vi "Set Data Value.vi"(8 "error in (no error)":errorcluster, 9 "Flat Data":u8[](array[numeric]) format="%.0x", 11 "CIFTag in":refnum<class "CIF_CIPC_Chn_String.lvclass">) -> (0 "error out":errorcluster, 1 "Updated":bool, 3 "CIFTag out":refnum<class "CIF_CIPC_Chn_String.lvclass">)   [LabVIEW 2021, in "CIF_CIPC_Chn_String.lvclass"]
uses:
  CIF_CIPC_Chn_String.lvclass
  CIF_CIPC_Chn_String.lvclass/CIF_CIPC_Chn_String.ctl
  <vilib>/CIF Foundation/CIF Utilities/Errors/Append Error Location.vi
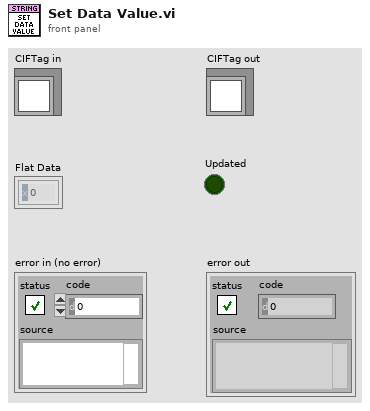
[diagram p1: front panel]
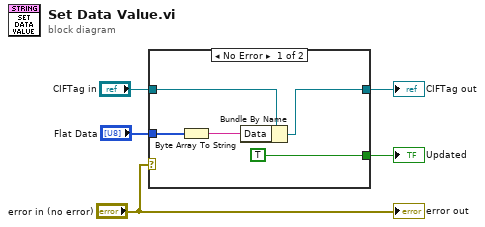
[diagram p0: block diagram]
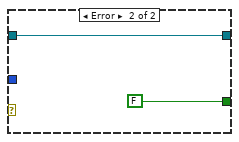
[diagram p2: hidden frame]
diagram:
  n1 = case shown="No Error" "error in (no error)" {
    tunnel: "Flat Data" -> [w7 _]
    tunnel: "CIFTag in" -> [w10 w12]
    tunnel: [w9 w12] -> w3
    tunnel: [TRUE FALSE] -> w2
    frame No Error {
      n2 = Byte Array To String(unsigned byte array=w7) -> (string=w6:string)
      n3 = Bundle By Name(cluster=w10, "Data"=w6) -> (w9:refnum<class "CIF_CIPC_Chn_String.lvclass">)
    }
    frame Error {
    }
  }
  "CIFTag out" <- w3
  "Updated" <- w2
  "error out" <- "error in (no error)"
